vi "TDMS Write Triggered Data.vi"() -> ()   [LabVIEW 2023]
doc: "Demonstrates how to write data from triggered measurements to a .tdms file with TDMS Write function."
uses:
  <vilib>/Utility/TDMS File Viewer/NI_TDMS File Viewer.lvlib
panel:
  in  "Trigger":bool
  in  "Stop":bool
  out "Number of Triggers":i32
  out "Measured Data":waveform(dbl)[](graph)
  # "Overview: Demonstrates how to write data from triggered measurements to a .tdms file with the TDMS Write function.\nInstructions:\n1. Run the VI.\n2. Click the Trigger button several times to write triggered data to the file.\n3. Click Stop to stop the VI.\n4. Delete the .tdms file (located at [LabVIEW Data]\\Example Triggered Data.tdms) when you are done."
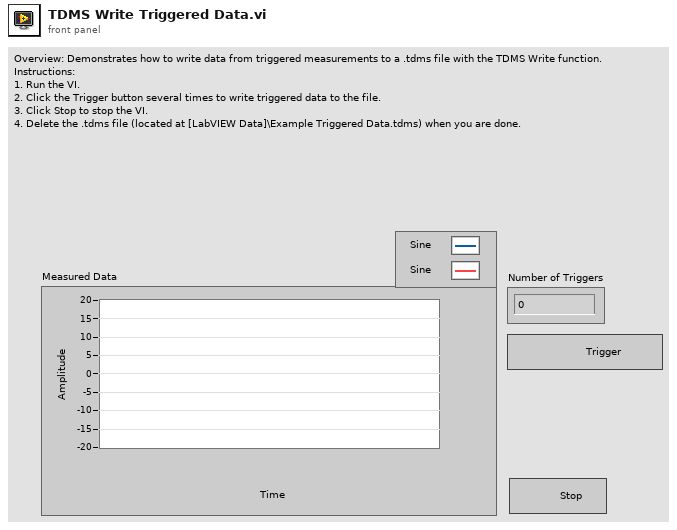
[diagram p1: front panel]
types:
  T1 = enum16{"open", "open or create", "create or replace", "create", "open (read-only)"}
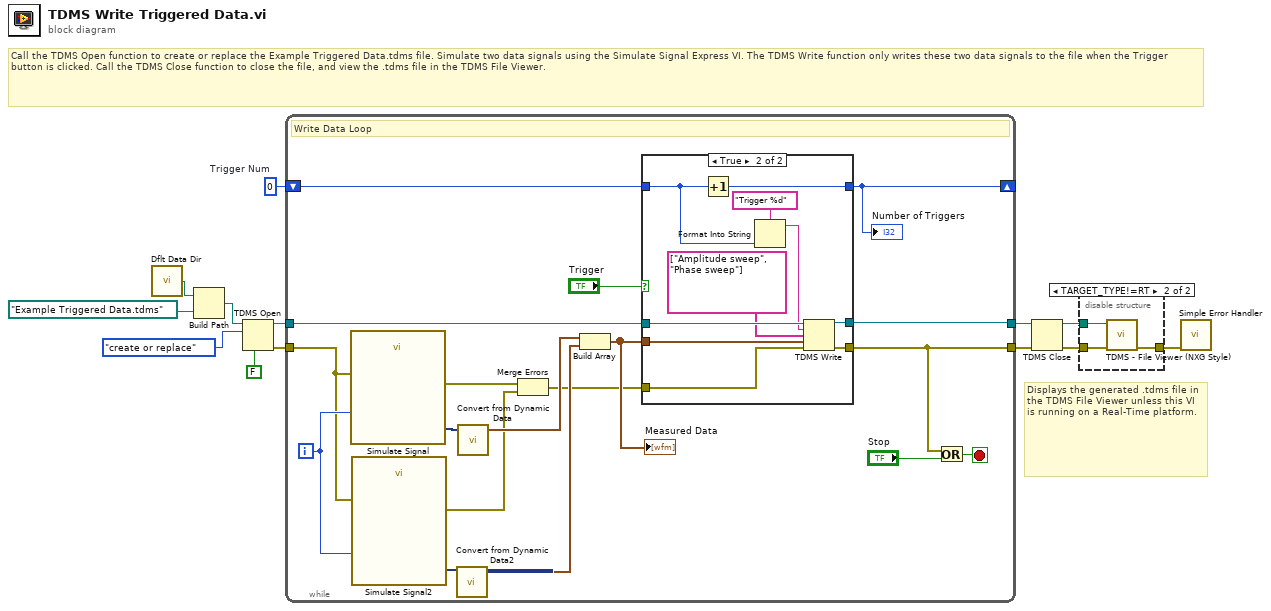
[diagram p0: block diagram]
diagram:
  w6 = 0  # Trigger Num
  # "Call the TDMS Open function to create or replace the Example Triggered Data.tdms file. Simulate two data signals using the Simulate Signal Express VI. The TDMS Write function only writes these two data signals to the file when the Trigger button is clicked. Call the TDMS Close function to close the file, and view the .tdms file in the TDMS File Viewer."
  # "Displays the generated .tdms file in the TDMS File Viewer unless this VI is running on a Real-Time platform."
  n1 = call <vilib>:"Dflt Data Dir.vi"() -> ("App:Default Data Directory"=w13:path)
  n2 = Build Path(base path=w13, name or relative path=path "Example Triggered Data.tdms" ("file path")) -> (appended path=w3:path)
  n3 = TDMS Open(6:FALSE ("disable buffering (T)"), 10:T1."create or replace" ("operation"), 11:w3) -> (0:w7:errorcluster, 3:w8:refnum<k34>)  [unwired: 4 in]
  n4 = while {
    shift-right: [w27] -> _
    shift-left: w6 -> [w28]
    tunnel: w8 -> [w31]
    tunnel: [w29] -> w10
    tunnel: w7 -> [w16]
    tunnel: [w24] -> w9
    i -> [w17]
    stop <- w26 stop-if-true
    # "Write Data Loop"
    n5 = call "Simulate Signal"("Amplitude"=w17, "error in (no error)"=w16) -> ("Sine"=w22:dynamicdata, "error out"=w14:errorcluster)  [unwired: 12 in]
    n6 = call "Simulate Signal2"("Phase"=w17, "error in (no error)"=w16) -> ("Sine"=w21:dynamicdata, "error out"=w18:errorcluster)  [unwired: 12 in]
    n7 = call "Convert from Dynamic Data2"("Dynamic Data Type"=w21) -> ("Waveform"=w20:waveform(dbl))  [unwired: 3 in]
    n8 = call "Convert from Dynamic Data"("Dynamic Data Type"=w22) -> ("Waveform"=w19:waveform(dbl))  [unwired: 3 in]
    n9 = Merge Errors(w14, w18) -> (w15:errorcluster)
    n10 = Build Array(w19, w20) -> (w30:waveform(dbl)[])
    "Measured Data" <- w30
    n11 = case shown="True" "Trigger" {
      tunnel: w31 -> [w34 w44]
      tunnel: w15 -> [w33 w43]
      tunnel: w30 -> [_ w41]
      tunnel: [w33 w40] -> w24
      tunnel: [w34 w39] -> w29
      tunnel: w28 -> [w32 w36]
      tunnel: [w32 w35] -> w27
      frame False {
      }
      frame True {
        n12 = Increment(x=w36) -> (x+1=w35:i32)
        n13 = Format Into String(format string="Trigger %d" ("group name"), w36) -> (resulting string=w37:string)  [unwired: 2 in, 1 out]
        n14 = TDMS Write(0:w44, 5:w37, 7:string[] ["Amplitude sweep", "Phase sweep"] ("channel names"), 9:w41, 11:w43) -> (4:w39:refnum<k34>, 15:w40:errorcluster)  [unwired: 1 in, 2 out]
      }
    }
    "Number of Triggers" <- w27
    n15 = Or(x=w24, y="Stop") -> (x .or. y?=w26:bool)
  }
  n16 = TDMS Close(8:w9, 11:w10) -> (0:w5:errorcluster, 3:w2:path)
  n17 = disable-structure shown="TARGET_TYPE!=RT" {
    disable-tunnel: w5 -> [w45 w48]
    disable-tunnel: w2 -> [_ w47]
    disable-tunnel: [w45 w46] -> w1
    frame condition #0 {
    }
    frame condition #1 (active) {
      n18 = call <vilib>:"TDMS - File Viewer (NXG Style).vi"("error in"=w48, "file in"=w47) -> ("error out"=w46:errorcluster)  [unwired: 8 in, 1 out]
    }
  }
  n19 = call <vilib>:"Simple Error Handler.vi"("error in (no error)"=w1) -> ()  [unwired: 2 in, 7 out]
